vi "Motor_GetFrictCompVol.vi"(8 "error in (no error)":errorcluster, 11 "MC_EC60f in":refnum<class "MC_EC60f.lvclass">) -> (0 "error out":errorcluster, 2 "FrictionVol":dbl[](array[numeric]), 3 "MC_EC60f out":refnum<class "MC_EC60f.lvclass">)   [LabVIEW 2014, in "MC_EC60f.lvclass"]
uses:
  MC_EC60f.lvclass
  MC_EC60f.lvclass/MC_EC60f.ctl
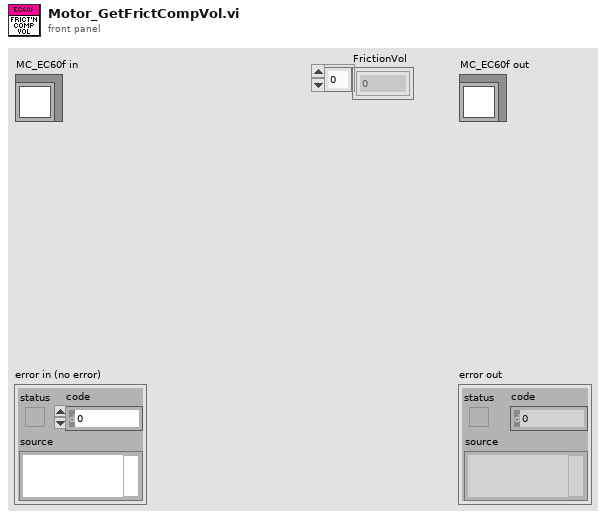
[diagram p1: front panel]
types:
  T1 = cluster{"Positive":cluster{"a":dbl, "b":dbl, "c":dbl}, "Negative":cluster{"a":dbl, "b":dbl, "c":dbl}}
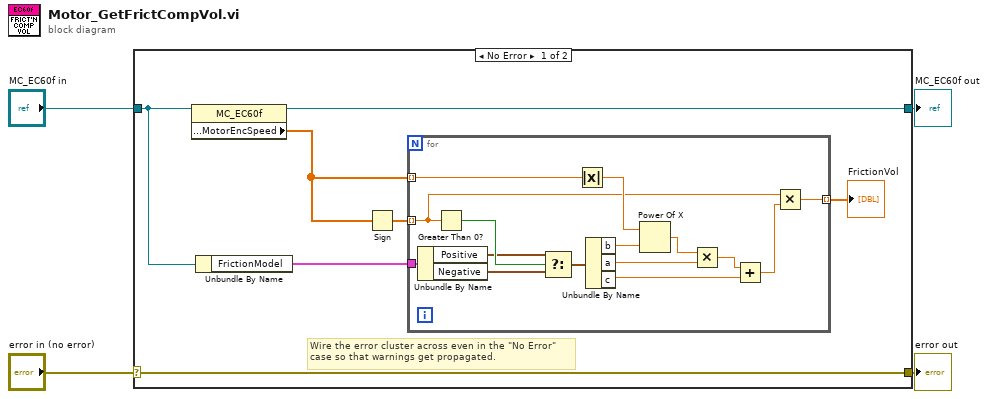
[diagram p0: block diagram]
diagram:
  n1 = case shown="No Error" "error in (no error)" {
    selector: "error in (no error)" -> [w11 w28]
    tunnel: [w11 w28] -> w3
    tunnel: [w9 w27] -> w1
    tunnel: "MC_EC60f in" -> [w10 w27]
    frame No Error {
      # "Wire the error cluster across even in the \"No Error\"\ncase so that warnings get propagated."
      n2 = property class="MC_EC60f"(reference=w10) -> (reference out=w9:refnum<class "MC_EC60f.lvclass">, "PropertyNode:MotorEncSpeed"=w8:dbl[])  [unwired: 1 in, 1 out]
      n3 = Unbundle By Name(w10) -> ("FrictionModel"=w7:T1)
      n4 = Sign(1:w8) -> (0:w6:dbl[])
      n5 = for {
        tunnel: w8 -> [w21] mode=indexing
        tunnel: w7 -> [w25]
        tunnel: w6 -> [w12] mode=indexing
        tunnel: [w13] -> w5 mode=indexing
        n6 = Unbundle By Name(w25) -> ("Positive"=w24:cluster{"a":dbl, "b":dbl, "c":dbl}, "Negative"=w23:cluster{"a":dbl, "b":dbl, "c":dbl})
        n7 = Greater Than 0?(x=w12) -> (x > 0?=w26:bool)
        n8 = Select(t=w24, s=w26, f=w23) -> (s? t:f=w22:cluster{"a":dbl, "b":dbl, "c":dbl})
        n9 = Absolute Value(x=w21) -> (abs(x)=w20:dbl)
        n10 = Unbundle By Name(w22) -> ("b"=w19:dbl, "a"=w17:dbl, "c"=w15:dbl)
        n11 = Power Of X(1:w19, 2:w20) -> (0:w18:dbl)
        n12 = Multiply(x=w18, y=w17) -> (x*y=w16:dbl)
        n13 = Add(x=w16, y=w15) -> (x+y=w14:dbl)
        n14 = Multiply(x=w12, y=w14) -> (x*y=w13:dbl)
      }
      "FrictionVol" <- w5
    }
    frame Error {
    }
  }
  "error out" <- w3
  "MC_EC60f out" <- w1
